vi "Memory.Pointer.Write Bytes.Unsafe.vi"(8 "error in (no error)":errorcluster, 9 "offset (0)":u64 format="%d bytes", 10 "buffer":u8[](array[numeric]) format="%02x", 11 "Pointer in":refnum<class "Memory.Pointer.Void.lvclass">) -> (0 "error out":errorcluster, 1 "offset dup":u64 format="%d bytes", 2 "buffer dup":u8[](array[numeric]) format="%02x", 3 "Pointer out":refnum<class "Memory.Pointer.Void.lvclass">)   [LabVIEW 2016, in "LabVIEW Memory Manager.lvlib" / "Memory.Pointer.Void.lvclass"]
uses:
  Memory.Pointer.Void.lvclass
  Memory.Pointer.Void.lvclass/Memory.Pointer.Void.ctl
  Memory.Pointer.Offset to Address.Unsafe.vi
  Memory.Pointer.Get Address.vi
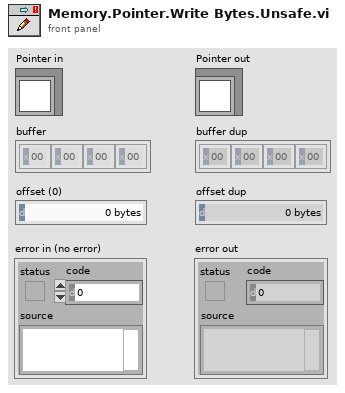
[diagram p1: front panel]
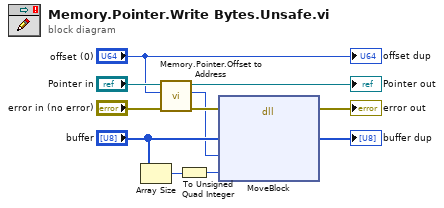
[diagram p0: block diagram]
diagram:
  n1 = Array Size(array="buffer") -> (size(s)=w3:i32)
  n2 = call-poly "Memory.Pointer.Offset to Address.vi"("error in (no error)"="error in (no error)", "offset"="offset (0)", "Pointer in"="Pointer in") -> ("error out"=w8:errorcluster, "address"=w1:u64, "Pointer out"=→"Pointer out":refnum<class "Memory.Pointer.Void.lvclass">)  [unwired: 6 in]
  n3 = To Unsigned Quad Integer(1:w3) -> (0:w2:u64)
  n4 = dll-call lib="LabVIEW" fn="MoveBlock"(error in=w8, "src pointer"="buffer", "dst pointer"=w1, "size"=w2) -> (error out=→"error out":errorcluster, "src pointer"=→"buffer dup":u8[])  [unwired: 5 in, 1 out]
  "offset dup" <- "offset (0)"
